vi "Grid_Scan_Stiching_V1.vi"() -> ()   [LabVIEW 2014]
uses:
  shared/CorrelImages (SubVI)Single.vi
  <userlib>/Nanonis Prog Interface V5/Nanonis Prog Interface.lvlib
panel:
  out "Current Coordinate":cluster{"Xc":sgl, "Yc":sgl} {"Yc" format="%.2p"; "Xc" format="%.2p"}
  out "Grid Coordinates":dbl[][](array[numeric])
  in  "img delay (s)":u32=1
  in  "TipLift (m)":sgl format="%#_6p"
  out "timing":i32
  out "Grid Size":cluster{"Width":sgl, "Height":sgl}
  out "Angle (deg)":sgl format="%.2f"
  out "Size (m)":cluster{"Width":sgl, "Height":sgl} {"Height" format="%.2p"; "Width" format="%.2p"}
  out "Center coordinates (m)":cluster{"Xc":sgl, "Yc":sgl} {"Yc" format="%.2p"; "Xc" format="%.2p"}
  in  "# of Grids":i32=1 min=1 max=10
  in  "ref bias":dbl=-0.0012 format="%#_6p"
  out "DC active":bool
  out "Y drift":sgl
  out "X drift":sgl
  in  "Current":dbl=5e-11 format="%#_6p"
  in  "Bias":dbl=0.02 format="%#_6p"
  in  "Settling time (s)":dbl=0.7 format="%#_6p"
  in  "Channel index (0-23)":u8(ring) items=["Current"=0, "Z (m)"=14]
  in  "Img Speed":sgl=4.5e-08 format="%#_6p"
  in  "Img Bias (V) DC":sgl=1.0 format="%_2p"
  in  "Img Current":sgl=1e-10 format="%#_6p"
  in  "Drift correction Pixels":i32=128
  in  "Forward Speed":sgl=1.2e-09 format="%#_6p"
  in  "Backward Speed":sgl=8e-08 format="%#_6p"
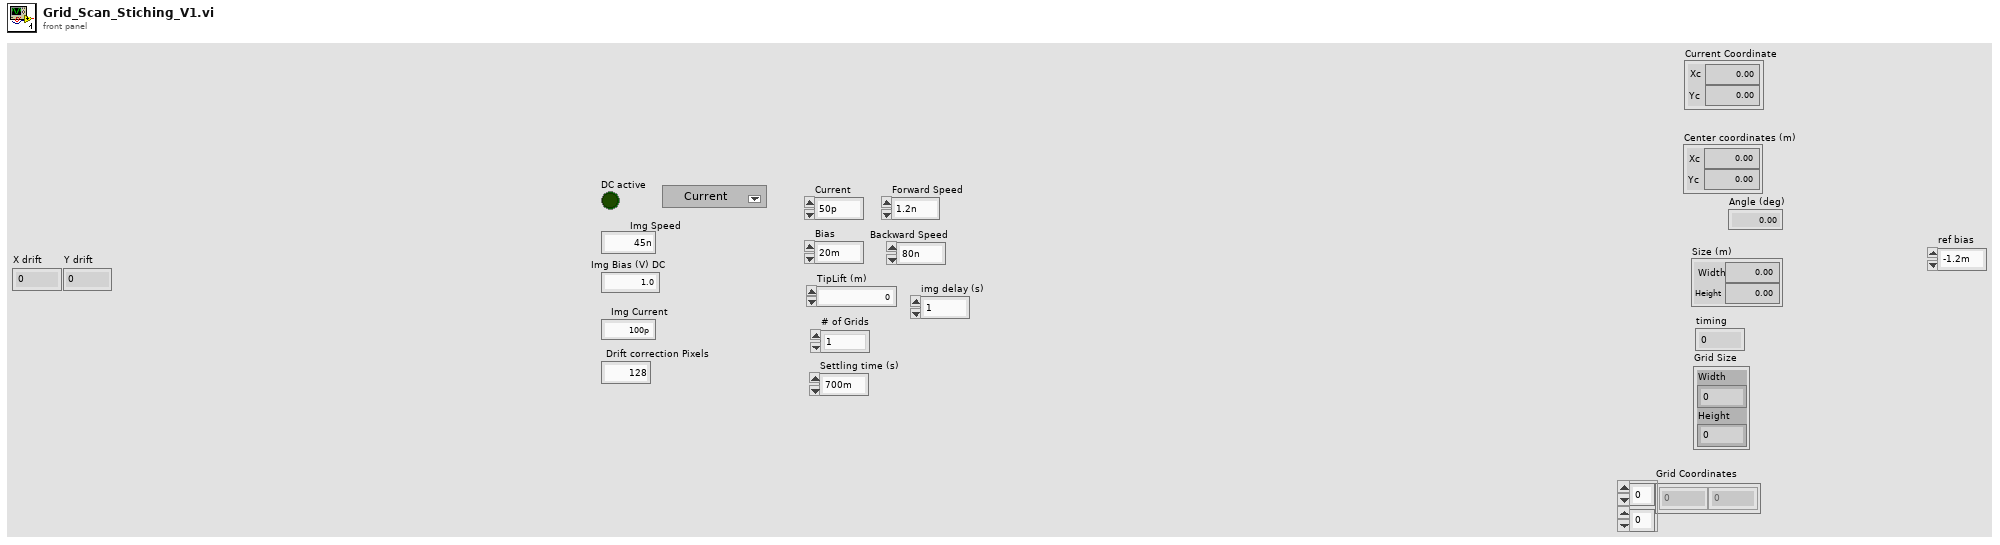
[diagram p1: front panel]
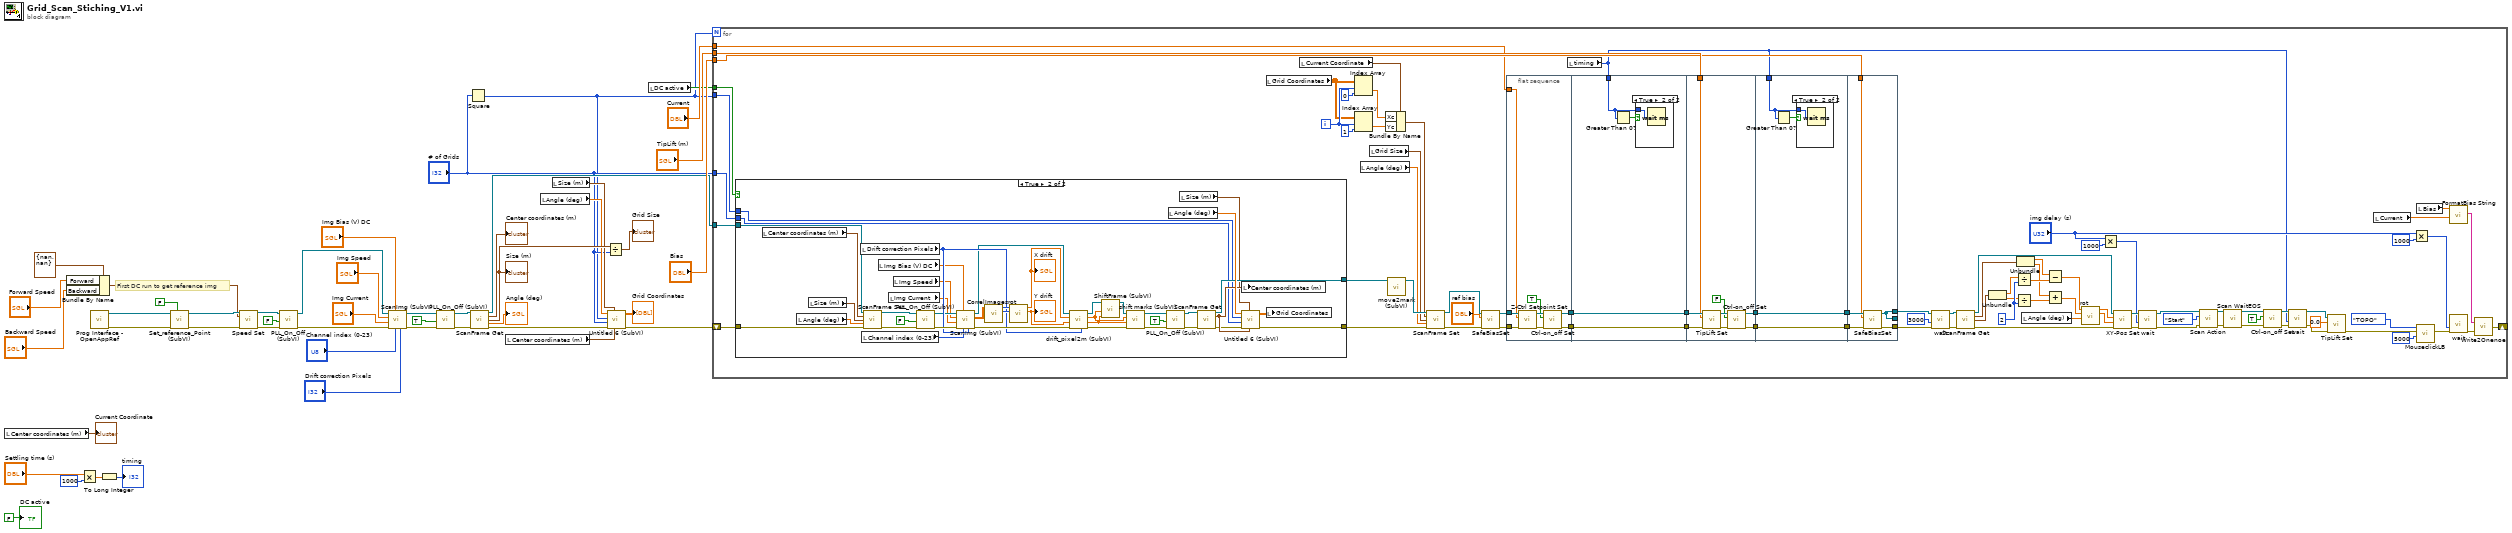
[diagram p0: block diagram]
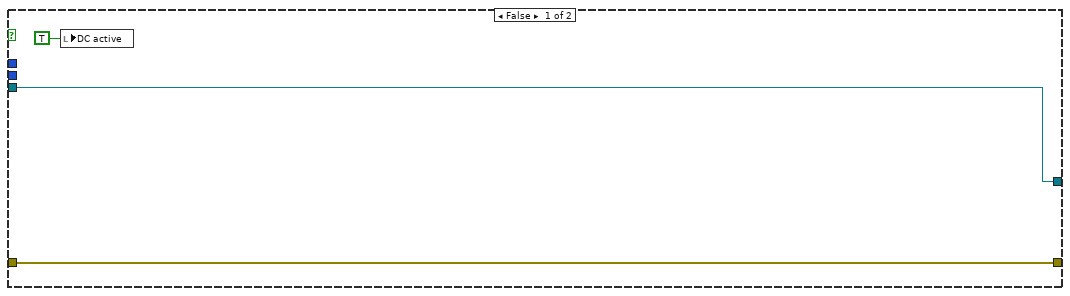
[diagram p2: hidden frame]
diagram:
  # "First DC run to get reference img"
  n1 = local read "Center coordinates (m)"() -> (→"Current Coordinate":cluster{"Xc":sgl, "Yc":sgl})
  n2 = Bundle By Name(cluster=cluster{"Forward":sgl, "Backward":sgl} {"Forward"=nan, "Backward"=nan} ("Speed (m/s)"), "Forward"="Forward Speed", "Backward"="Backward Speed") -> (w40:cluster{"Forward":sgl, "Backward":sgl})
  n3 = Multiply(x="Settling time (s)", y=u32 1000) -> (x*y=w21:dbl)
  n4 = call <userlib>:"Prog Interface - OpenAppRef.vi"() -> ("Error out"=w46:errorcluster, "Application reference"=w47:refnum<vi>)  [unwired: 6 in]
  n5 = To Long Integer(number=w21) -> (32bit integer=→"timing":i32)
  n6 = call "Set_reference_Point (SubVI).vi"("Part of multigrid"=FALSE, "error in (no error)"=w46, "Application in"=w47) -> ("error out"=w42:errorcluster, "Application out"=w41:refnum<vi>)  [unwired: 7 in]
  n7 = call <userlib>:"Speed Set.vi"("Application ref in"=w41, "Speed (m/s)"=w40, "error in (no error)"=w42) -> ("Application ref out"=w37:refnum<vi>, "error out"=w38:errorcluster)  [unwired: 11 in]
  n8 = call "PLL_On_Off (SubVI).vi"("error in (no error)"=w38, "Output ON/OFF (F=OFF)"=FALSE, "Application in"=w37) -> ("error out"=w29:errorcluster, "Application out"=w30:refnum<vi>)  [unwired: 7 in]
  n9 = call "ScanImg (SubVI).vi"("pixel"="Drift correction Pixels", "Channel index (0-23)"="Channel index (0-23)", "Bias (V)"="Img Bias (V) DC", "error in (no error)"=w29, "Current"="Img Current", "Img Speed"="Img Speed", "Application in"=w30) -> ("error out"=w33:errorcluster, "Application out"=w34:refnum<vi>)  [unwired: 2 in, 1 out]
  n10 = call "PLL_On_Off (SubVI).vi"("error in (no error)"=w33, "Output ON/OFF (F=OFF)"=TRUE, "Application in"=w34) -> ("error out"=w25:errorcluster, "Application out"=w26:refnum<vi>)  [unwired: 7 in]
  n11 = Square(x="# of Grids") -> (x^2=w2:i32)
  n12 = call <userlib>:"ScanFrame Get.vi"("Application ref in"=w26, "error in (no error)"=w25) -> ("Application ref out"=w4:refnum<vi>, "Center coordinates (m)"=→"Center coordinates (m)":cluster{"Xc":sgl, "Yc":sgl}, "Size (m)"=w17:cluster{"Width":sgl, "Height":sgl}, "Angle (deg)"=→"Angle (deg)":sgl, "error out"=w8:errorcluster)  [unwired: 9 in]
  "Size (m)" <- w17
  n13 = local read "Center coordinates (m)"() -> (w12:cluster{"Xc":sgl, "Yc":sgl})
  n14 = local read "Angle (deg)"() -> (w9:sgl)
  n15 = local read "Size (m)"() -> (w11:cluster{"Width":sgl, "Height":sgl})
  n16 = Divide(x=w17, y="# of Grids") -> (x/y=→"Grid Size":cluster{"Width":sgl, "Height":sgl})
  n17 = call "Untitled 6 (SubVI).vi"("Center coordinates (m)"=w12, "Size (m)"=w11, "error in (no error)"=w8, "# of Grids"="# of Grids", "Numeric"=w2, "Angle (deg)"=w9) -> ("error out"=w6:errorcluster, "Array"=→"Grid Coordinates":sgl[][])  [unwired: 4 in]
  n18 = local read "DC active"() -> (w5:bool)
  n19 = for {
    N: w2 -> [_]
    tunnel: "TipLift (m)" -> [w121]
    tunnel: "Bias" -> [w120]
    shift-right: [w56] -> _
    shift-left: w6 -> [w53]
    tunnel: "Current" -> [w55]
    tunnel: w5 -> [w52]
    tunnel: w4 -> [w50]
    tunnel: "# of Grids" -> [w49]
    tunnel: w2 -> [w48]
    i -> [w77]
    w102 = 2
    n20 = case shown="True" w52 {
      tunnel: [w134 w145] -> w54
      tunnel: w53 -> [w134 w142]
      tunnel: [w133 w150] -> w51
      tunnel: w50 -> [w133 w141]
      tunnel: w49 -> [_ w144]
      tunnel: w48 -> [_ w143]
      frame False {
        n21 = local write "DC active"(TRUE ("DC active")) -> ()
      }
      frame True {
        n22 = local read "Center coordinates (m)"() -> (w138:cluster{"Xc":sgl, "Yc":sgl})
        n23 = local read "Angle (deg)"() -> (w136:sgl)
        n24 = local read "Size (m)"() -> (w137:cluster{"Width":sgl, "Height":sgl})
        n25 = local read "Drift correction Pixels"() -> (w170:i32)
        n26 = local read "Channel index (0-23)"() -> (w165:u8)
        n27 = call <userlib>:"ScanFrame Set.vi"("Application ref in"=w141, "Center coordinates (m)"=w138, "Size (m)"=w137, "Angle (deg)"=w136, "error in (no error)"=w142) -> ("Application ref out"=w140:refnum<vi>, "error out"=w139:errorcluster)  [unwired: 9 in]
        n28 = local read "Img Bias (V) DC"() -> (w164:sgl)
        n29 = local read "Img Current"() -> (w163:sgl)
        n30 = local read "Img Speed"() -> (w162:sgl)
        n31 = call "PLL_On_Off (SubVI).vi"("error in (no error)"=w139, "Output ON/OFF (F=OFF)"=FALSE, "Application in"=w140) -> ("error out"=w175:errorcluster, "Application out"=w168:refnum<vi>)  [unwired: 7 in]
        n32 = call "ScanImg (SubVI).vi"("pixel"=w170, "Channel index (0-23)"=w165, "Bias (V)"=w164, "error in (no error)"=w175, "Current"=w163, "Img Speed"=w162, "Application in"=w168) -> ("error out"=w176:errorcluster, "Img"=w161:dbl[][], "Application out"=w167:refnum<vi>)  [unwired: 2 in]
        n33 = call-poly "CorrelImages.vi"("New Image"=w161) -> ("Y drift"=w173:i32, "X drift"=w171:i32)  [unwired: 7 in, 2 out]
        n34 = call "rot.vi"("y"=w173, "x"=w171) -> ("y'"=w174:sgl, "x'"=w172:sgl)  [unwired: 8 in]
        "X drift" <- w172
        "Y drift" <- w174
        n35 = call "drift_pixel2m (SubVI).vi"("Application in"=w167, "X drift"=w172, "Y drift"=w174, "error in"=w176, "Drift correction Pixels"=w170) -> ("Application out"=w166:refnum<vi>, "x drift"=w159:sgl, "y drift"=w158:sgl, "error out"=w157:errorcluster)  [unwired: 1 in]
        n36 = call "ShiftFrame (SubVI).vi"("Y shift"=w158, "X shift"=w159, "Application in"=w166) -> ("Application out"=w160:refnum<vi>)  [unwired: 8 in]
        n37 = call "shift marks (SubVI).vi"("error in (no error)"=w157, "y"=w158, "x"=w159, "Application in"=w160) -> ("error out"=w155:errorcluster, "Application out"=w156:refnum<vi>)  [unwired: 6 in]
        n38 = call "PLL_On_Off (SubVI).vi"("error in (no error)"=w155, "Output ON/OFF (F=OFF)"=TRUE, "Application in"=w156) -> ("error out"=w151:errorcluster, "Application out"=w152:refnum<vi>)  [unwired: 7 in]
        n39 = local read "Angle (deg)"() -> (w153:sgl)
        n40 = local read "Size (m)"() -> (w148:cluster{"Width":sgl, "Height":sgl})
        n41 = call <userlib>:"ScanFrame Get.vi"("Application ref in"=w152, "error in (no error)"=w151) -> ("Application ref out"=w150:refnum<vi>, "Center coordinates (m)"=w149:cluster{"Xc":sgl, "Yc":sgl}, "error out"=w146:errorcluster)  [unwired: 9 in, 2 out]
        n42 = local write "Center coordinates (m)"(w149) -> ()
        n43 = call "Untitled 6 (SubVI).vi"("Center coordinates (m)"=w149, "Size (m)"=w148, "error in (no error)"=w146, "# of Grids"=w144, "Numeric"=w143, "Angle (deg)"=w153) -> ("error out"=w145:errorcluster, "Array"=w147:sgl[][])  [unwired: 4 in]
        n44 = local write "Grid Coordinates"(w147) -> ()
      }
    }
    n45 = local read "Grid Coordinates"() -> (w73:dbl[][])
    n46 = local read "Current Coordinate"() -> (w72:cluster{"Xc":sgl, "Yc":sgl})
    n47 = Index Array(array=w73, index (row)=w77, index (col)=0 ("disabled index (col)")) -> (element=w74:dbl)
    n48 = Index Array(array=w73, index (row)=w77, index (col)=1) -> (element=w71:dbl)
    n49 = local read "Angle (deg)"() -> (w68:sgl)
    n50 = local read "Grid Size"() -> (w69:cluster{"Width":sgl, "Height":sgl})
    n51 = Bundle By Name(cluster=w72, "Xc"=w74, "Yc"=w71) -> (w70:cluster{"Xc":sgl, "Yc":sgl})
    n52 = call "move2mark (SubVI).vi"("Application in"=w51) -> ("Application out"=w80:refnum<vi>)  [unwired: 10 in]
    n53 = call <userlib>:"ScanFrame Set.vi"("Application ref in"=w80, "Center coordinates (m)"=w70, "Size (m)"=w69, "Angle (deg)"=w68, "error in (no error)"=w54) -> ("Application ref out"=w79:refnum<vi>, "error out"=w78:errorcluster)  [unwired: 9 in]
    n54 = call "SafeBiasSet.vi"("Application ref in"=w79, "Bias (V)"="ref bias", "error in (no error)"=w78) -> ("Application ref out"=w123:refnum<vi>, "Error out"=w124:errorcluster)  [unwired: 6 in]
    n55 = flat-sequence {
      tunnel: [w183] -> w132
      tunnel: [w180] -> w131
      tunnel: w123 -> [w179]
      tunnel: w124 -> [w178]
      tunnel: w55 -> [w177]
      tunnel: w132 -> [w188]
      tunnel: [w188] -> w130
      tunnel: w83 -> [w186]
      tunnel: [w185] -> w129
      tunnel: w131 -> [w185]
      tunnel: w130 -> [w197]
      tunnel: [w195] -> w128
      tunnel: w129 -> [w194]
      tunnel: [w192] -> w127
      tunnel: w121 -> [w190]
      tunnel: w128 -> [w201]
      tunnel: [w201] -> w126
      tunnel: [w199] -> w125
      tunnel: w127 -> [w199]
      tunnel: w83 -> [w198]
      tunnel: [w203] -> _
      tunnel: w126 -> [w207]
      tunnel: w125 -> [w206]
      tunnel: [w205] -> w82
      tunnel: w120 -> [w204]
      tunnel: [w203] -> w81
      frame #0 {
        n56 = call <userlib>:"Z-Ctrl Setpoint Set.vi"("error in (no error)"=w178, "Z Controller setpoint"=w177, "Application ref in"=w179) -> ("error out"=w181:errorcluster, "Application ref out"=w184:refnum<vi>)  [unwired: 7 in]
        n57 = call <userlib>:"Ctrl-on_off Set.vi"("error in (no error)"=w181, "Z Controller ON/OFF"=TRUE, "Application ref in"=w184) -> ("error out"=w180:errorcluster, "Application ref out"=w183:refnum<vi>)  [unwired: 7 in]
      }
      frame #1 {
        n58 = Greater Than 0?(x=w186) -> (x > 0?=w187:bool)
        n59 = case shown="True" w187 {
          tunnel: w186 -> [_ w189]
          frame False {
          }
          frame True {
            n60 = Wait (ms)(milliseconds to wait=w189) -> ()  [unwired: 1 out]
          }
        }
      }
      frame #2 {
        n61 = call <userlib>:"TipLift Set.vi"("error in (no error)"=w194, "TipLift (m)"=w190, "Application ref in"=w197) -> ("error out"=w193:errorcluster, "Application ref out"=w196:refnum<vi>)  [unwired: 7 in]
        n62 = call <userlib>:"Ctrl-on_off Set.vi"("error in (no error)"=w193, "Z Controller ON/OFF"=FALSE, "Application ref in"=w196) -> ("error out"=w192:errorcluster, "Application ref out"=w195:refnum<vi>)  [unwired: 7 in]
      }
      frame #3 {
        n63 = Greater Than 0?(x=w198) -> (x > 0?=w200:bool)
        n64 = case shown="True" w200 {
          tunnel: w198 -> [_ w202]
          frame False {
          }
          frame True {
            n65 = Wait (ms)(milliseconds to wait=w202) -> ()  [unwired: 1 out]
          }
        }
      }
      frame #4 {
        n66 = call "SafeBiasSet.vi"("Application ref in"=w207, "Bias (V)"=w204, "error in (no error)"=w206) -> ("Application ref out"=w203:refnum<vi>, "Error out"=w205:errorcluster)  [unwired: 6 in]
      }
    }
    n67 = local read "timing"() -> (w83:i32)
    n68 = call "wait.vi"("error in"=w82, "milliseconds to wait"=u32 3000 ("y"), "application reference in"=w81) -> ("error out"=w94:errorcluster, "application reference out"=w93:refnum<vi>)  [unwired: 7 in]
    n69 = call <userlib>:"ScanFrame Get.vi"("Application ref in"=w93, "error in (no error)"=w94) -> ("Application ref out"=w111:refnum<vi>, "Center coordinates (m)"=w97:cluster{"Xc":sgl, "Yc":sgl}, "Size (m)"=w98:cluster{"Width":sgl, "Height":sgl}, "error out"=w110:errorcluster)  [unwired: 9 in, 1 out]
    n70 = Unbundle(w98) -> ("Width"=w100:sgl, "Height"=w101:sgl)
    n71 = Divide(x=w100, y=w102) -> (x/y=w104:sgl)
    n72 = Divide(x=w101, y=w102) -> (x/y=w103:sgl)
    n73 = Unbundle(w97) -> ("Xc"=w105:sgl, "Yc"=w99:sgl)
    n74 = local read "Angle (deg)"() -> (w65:sgl)
    n75 = Subtract(x=w105, y=w104) -> (x-y=w67:sgl)
    n76 = Add(x=w99, y=w103) -> (x+y=w66:sgl)
    n77 = call "rot.vi"("angle"=w65, "y"=w66, "x"=w67) -> ("y'"=w63:sgl, "x'"=w64:sgl)  [unwired: 7 in]
    n78 = Multiply(x="img delay (s)", y=u32 1000) -> (x*y=w107:u32)
    n79 = call <userlib>:"XY-Pos Set.vi"("error in (no error)"=w110, "Y (m)"=w63, "X (m)"=w64, "Application ref in"=w111) -> ("error out"=w109:errorcluster, "Application ref out"=w108:refnum<vi>)  [unwired: 4 in]
    n80 = call "wait.vi"("error in"=w109, "milliseconds to wait"=w107, "application reference in"=w108) -> ("error out"=w91:errorcluster, "application reference out"=w92:refnum<vi>)  [unwired: 7 in]
    n81 = call <userlib>:"Scan Action.vi"("error in (no error)"=w91, "Scan action (Start)"=enum16{"Start", "Stop", "Pause", "Resume"}."Start", "Application ref in"=w92) -> ("error out"=w89:errorcluster, "Application ref out"=w90:refnum<vi>)  [unwired: 6 in]
    n82 = call <userlib>:"Scan WaitEOS.vi"("error in (no error)"=w89, "Application ref in"=w90) -> ("error out"=w61:errorcluster, "Application ref out"=w62:refnum<vi>)  [unwired: 5 in, 2 out]
    n83 = call <userlib>:"Ctrl-on_off Set.vi"("error in (no error)"=w61, "Z Controller ON/OFF"=TRUE, "Application ref in"=w62) -> ("error out"=w87:errorcluster, "Application ref out"=w85:refnum<vi>)  [unwired: 7 in]
    n84 = call "wait.vi"("error in"=w87, "milliseconds to wait"=w83, "application reference in"=w85) -> ("error out"=w86:errorcluster, "application reference out"=w84:refnum<vi>)  [unwired: 7 in]
    n85 = call <userlib>:"TipLift Set.vi"("error in (no error)"=w86, "TipLift (m)"=sgl 0.0, "Application ref in"=w84) -> ("error out"=w118:errorcluster)  [unwired: 7 in, 1 out]
    n86 = local read "Current"() -> (w57:dbl)
    n87 = Multiply(x="img delay (s)", y=u32 1000) -> (x*y=w113:u32)
    n88 = call "MouseclickLB.vi"("nMilliseconds"=5000, "error in (no error)"=w118, "Click"=enum16{"Header", "TOPO", "STS", "GRID"}."TOPO") -> ("error out"=w112:errorcluster)  [unwired: 8 in]
    n89 = local read "Bias"() -> (w58:dbl)
    n90 = call "FormatBias String.vi"("current"=w57, "bias"=w58) -> ("resulting string"=w59:string)  [unwired: 9 in]
    n91 = call "wait.vi"("error in"=w112, "milliseconds to wait"=w113) -> ("error out"=w60:errorcluster)  [unwired: 8 in, 1 out]
    n92 = call "Write2Onenoe.vi"("error in (no error)"=w60, "strSendText"=w59) -> ("error out"=w56:errorcluster)
  }
  "DC active" <- FALSE ("DC active")
